vi "Build DashBoard Data.vi"(8 "OutputsCluster":T9, 10 "Command_Inputs":T1, 11 "Sensor_Inputs":T20) -> ()   [LabVIEW 2012]
doc: "This VI builds data and sends it back to the dashboard PC program. By default it sends back the raw values for the first analog, digital, and solenoid module. Modify it to send back the data you want to view. Consider adding higher level data to the Dashboard Datatype.ctl and to this VI. Then update the Dashboard to display the data however you like.\n\nThis software is licensed. Open the labview\\readme\\WPI Robotics Library Open Source License.txt file for more information."
uses:
  Dashboard Datatype.ctl
  Inputs_All.ctl
  Flywheel/Sensor_Inputs_FlyWheel.ctl
  tankdrive/Input_Sensors_Drive.ctl
  Conveyor/Sensor_Input_Conveyor.ctl
  Conveyor/Sensor_Input_ConveyorV2.ctl
  Turret/Inputs_Sensors_Turret.ctl
  Inputs_Camera.ctl
  Outputs_All.ctl
  Flywheel/Outputs_Flywheel.ctl
  tankdrive/Output_Wheel_Speeds.ctl
  Conveyor/Conveyor_outputs.ctl
  Conveyor/Conveyor module state.ctl
  Conveyor/Conveyor_outputsV2.ctl
  Conveyor/3-Ball-Conveyor_Module_State.ctl
  Conveyor/T_Roller module state.ctl
  Turret/Outputs_Turret.ctl
  Roller/Outputs_Roller.ctl
  Bridge Tipper/Outputs_Tipper.ctl
  Command_Inputs.ctl
  tankdrive/Input_Commands_Drive.ctl
  Conveyor/Input_Command_Conveyor.ctl
  Turret/Inputs_Commands_Turret.ctl
  Bridge Tipper/Inputs_Tipper.ctl
  Dashboard Controls.ctl
  Roller/Input_Commands_Roller.ctl
  Flywheel/Input_Commands_Flywheel.ctl
panel:
  out "error out":errorcluster
  out "Dashboard Data":T27
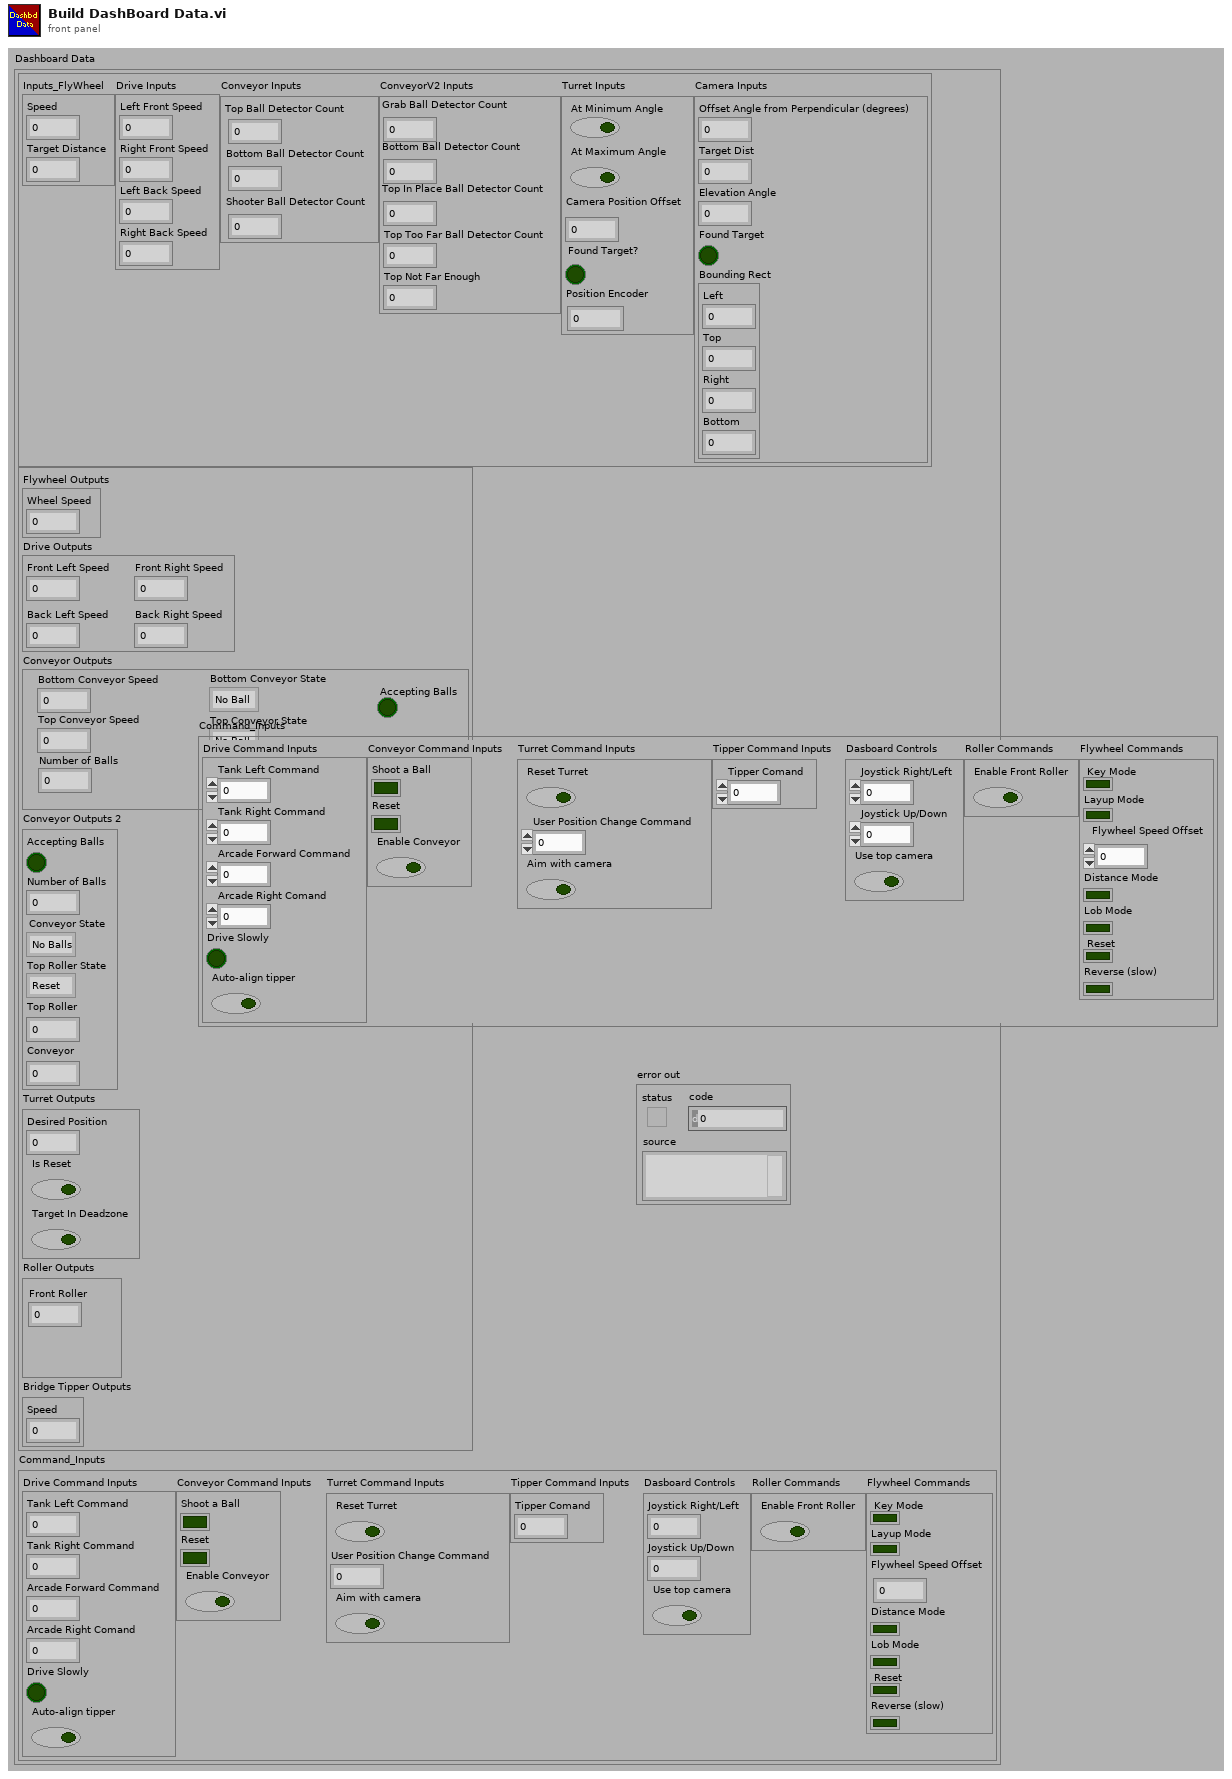
[diagram p1: front panel]
types:
  T1 = typedef "Command_Inputs.ctl" = cluster{"Drive Command Inputs":T2, "Conveyor Command Inputs":T3, "Turret Command Inputs":T4, "Tipper Command Inputs":T5, "Dasboard Controls":T6, "Roller Commands":T7, "Flywheel Commands":T8}
  T2 = typedef "Input_Commands_Drive.ctl" = cluster{"Tank Left Command":dbl, "Tank Right Command":dbl, "Arcade Forward Command":dbl, "Arcade Right Comand":dbl, "Drive Slowly":bool, "Auto-align tipper":bool}
  T3 = typedef "Input_Command_Conveyor.ctl" = cluster{"Shoot a Ball":bool, "Reset":bool, "Enable Conveyor":bool}
  T4 = typedef "Inputs_Commands_Turret.ctl" = cluster{"Reset Turret":bool, "User Position Change Command":dbl, "Aim with camera":bool}
  T5 = typedef "Inputs_Tipper.ctl" = cluster{"Tipper Comand":dbl}
  T6 = typedef "Dashboard Controls.ctl" = cluster{"Joystick Right/Left":dbl, "Joystick Up/Down":dbl, "Use top camera":bool}
  T7 = typedef "Input_Commands_Roller.ctl" = cluster{"Enable Front Roller":bool}
  T8 = typedef "Input_Commands_Flywheel.ctl" = cluster{"Key Mode":bool, "Layup Mode":bool, "Flywheel Speed Offset":dbl, "Distance Mode":bool, "Lob Mode":bool, "Reset":bool, "Reverse (slow)":bool}
  T9 = typedef "Outputs_All.ctl" = cluster{"Flywheel Outputs":T10, "Drive Outputs":T11, "Conveyor Outputs":T12, "Conveyor Outputs 2":T14, "Turret Outputs":T17, "Roller Outputs":T18, "Bridge Tipper Outputs":T19}
  T10 = typedef "Outputs_Flywheel.ctl" = cluster{"Wheel Speed":dbl}
  T11 = typedef "Output_Wheel_Speeds.ctl" = cluster{"Front Left Speed":dbl, "Front Right Speed":dbl, "Back Left Speed":dbl, "Back Right Speed":dbl}
  T12 = typedef "Conveyor_outputs.ctl" = cluster{"Bottom Conveyor Speed":dbl, "Top Conveyor Speed":dbl, "Bottom Conveyor State":T13, "Top Conveyor State":T13, "Accepting Balls":bool, "Number of Balls":i32}
  T13 = typedef "Conveyor module state.ctl" = enum16{"No Ball", "Has Ball", "Ball Below Hold", "Ball Above Hold", "Outputting Ball", "Reset"}
  T14 = typedef "Conveyor_outputsV2.ctl" = cluster{"Accepting Balls":bool, "Number of Balls":i32, "Conveyor State":T15, "Top Roller State":T16, "Top Roller":dbl, "Conveyor":dbl}
  T15 = typedef "3-Ball-Conveyor_Module_State.ctl" = enum16{"No Balls", "Collecting Ball", "Holding 1", "Pushing Ball Out", "Holding 2", "Lowering Ball", "Reset", "Disabled"}
  T16 = typedef "T_Roller module state.ctl" = enum16{"Reset", "Disabled", "Waiting for Ball", "Holding", "Ball not far enough", "Ball too far", "Firing"}
  T17 = typedef "Outputs_Turret.ctl" = cluster{"Desired Position":dbl, "Is Reset":bool, "Target In Deadzone":bool}
  T18 = typedef "Outputs_Roller.ctl" = cluster{"Front Roller":dbl}
  T19 = typedef "Outputs_Tipper.ctl" = cluster{"Speed":dbl}
  T20 = typedef "Inputs_All.ctl" = cluster{"Inputs_FlyWheel":T21, "Drive Inputs":T22, "Conveyor Inputs":T23, "ConveyorV2 Inputs":T24, "Turret Inputs":T25, "Camera Inputs":T26}
  T21 = typedef "Sensor_Inputs_FlyWheel.ctl" = cluster{"Speed":dbl, "Target Distance":dbl}
  T22 = typedef "Input_Sensors_Drive.ctl" = cluster{"Left Front Speed":dbl, "Right Front Speed":dbl, "Left Back Speed":dbl, "Right Back Speed":dbl}
  T23 = typedef "Sensor_Input_Conveyor.ctl" = cluster{"Top Ball Detector Count":i32, "Bottom Ball Detector Count":i32, "Shooter Ball Detector Count":i32}
  T24 = typedef "Sensor_Input_ConveyorV2.ctl" = cluster{"Grab Ball Detector Count":i32, "Bottom Ball Detector Count":i32, "Top In Place Ball Detector Count":i32, "Top Too Far Ball Detector Count":i32, "Top Not Far Enough":i32}
  T25 = typedef "Inputs_Sensors_Turret.ctl" = cluster{"At Minimum Angle":bool, "At Maximum Angle":bool, "Camera Position Offset":dbl, "Found Target?":bool, "Position Encoder":dbl}
  T26 = typedef "Inputs_Camera.ctl" = cluster{"Offset Angle from Perpendicular (degrees)":dbl, "Target Dist":dbl, "Elevation Angle":dbl, "Found Target":bool, "Bounding Rect":cluster{"Left":dbl, "Top":dbl, "Right":dbl, "Bottom":dbl}}
  T27 = typedef "Dashboard Datatype.ctl" = cluster{"Inputs_All":T20, "OutputsCluster":T9, "Command_Inputs":T1}
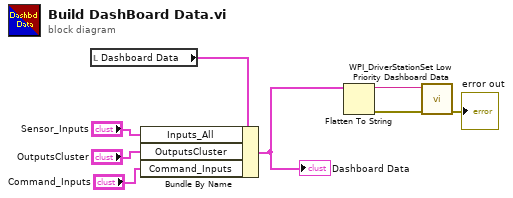
[diagram p0: block diagram]
diagram:
  n1 = local read "Dashboard Data"() -> (w8:T27)
  n2 = Bundle By Name(cluster=w8, "Inputs_All"="Sensor_Inputs", "OutputsCluster"="OutputsCluster", "Command_Inputs"="Command_Inputs") -> (w7:T27)
  "Dashboard Data" <- w7
  n3 = Flatten To String(anything=w7) -> (data string=w4:string, error out=w3:errorcluster)  [unwired: 1 in, 3 out]
  n4 = call <vilib>:"WPI_DriverStationSet Low Priority Dashboard Data.vi"("error in (no error)"=w3, "User Data"=w4) -> ("error out"=→"error out":errorcluster)  [unwired: 9 out]
